vi "Launch Soft Panel.vi"(8 "error in (no error)":errorcluster, 10 "SubPanel Ref":i32, 11 "Instrument in":refnum<class "Instrument.lvclass">) -> (0 "error out":errorcluster, 3 "Instrument out":refnum<class "Instrument.lvclass">)   [LabVIEW 2015, in "Instrument.lvlib" / "Instrument.lvclass"]
uses:
  Instrument.lvclass
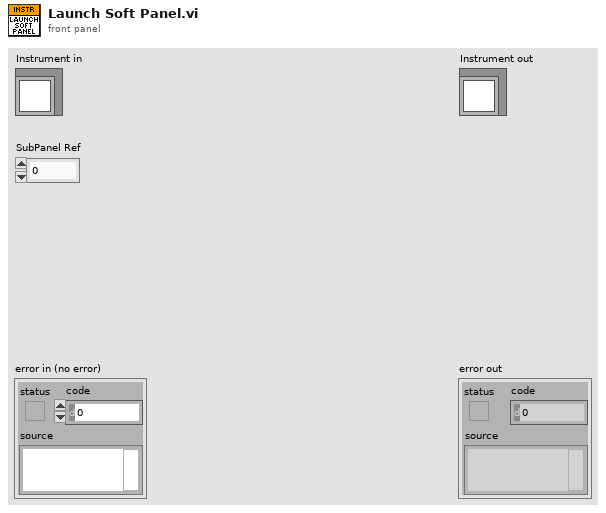
[diagram p1: front panel]
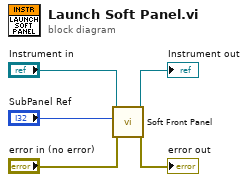
[diagram p0: block diagram]
diagram:
  n1 = call-dynamic "Soft Front Panel.vi"("error in (no error)"="error in (no error)", "SubPanel Ref"="SubPanel Ref", "Instrument in"="Instrument in") -> ("error out"=→"error out":errorcluster, "Instrument out"=→"Instrument out":refnum<class "Instrument.lvclass">)  [unwired: 7 in]
